vi "0036-Sub_save2.vi"   [LabVIEW 2014]
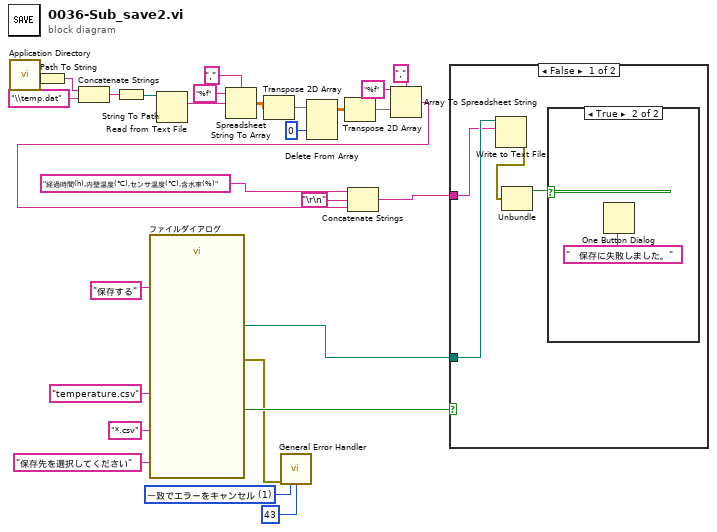
[diagram p0: block diagram]
diagram:
  w10 = 1 items=["例外なし", "一致でエラーをキャンセル", "一致でエラーをセット"] ("[exception action] (none:0)")
  n1 = call <vilib>:"Application Directory.vi"() -> ("Application Directory"=w2:path)
  n2 = Path To String(path=w2) -> (string=w3:string)
  n3 = Concatenate Strings(w3, "\\temp.dat" ("文字列")) -> (w4:string)
  n4 = String To Path(string=w4) -> (path=w5:path)
  n5 = call "ファイルダイアログ"("prompt"="保存先を選択してください", "button label"="保存する", "default name"="temperature.csv", "pattern (all files)"="*.csv") -> ("selected path"=w13:path, "cancelled"=w14:bool, "error out"=w12:errorcluster)  [unwired: 8 in, 1 out]
  n6 = Read from Text File(file (use dialog)=w5) -> (text=w15:string)  [unwired: 3 in, 3 out]
  n7 = Spreadsheet String To Array(delimiter (Tab)="," ("デリミタ（タブ）"), format string="%f" ("形式文字列"), spreadsheet string=w15) -> (array=w24:dbl[][])  [unwired: 1 in]
  n8 = Transpose 2D Array(2D array=w24) -> (transposed array=w18:dbl[][])
  n9 = call <vilib>:"General Error Handler.vi"("error in (no error)"=w12, "[exception action] (none:0)"=w10, "[exception code]"=43) -> ()  [unwired: 8 in, 5 out]
  n10 = Delete From Array(array=w18, index (row)=0 ("指標 （行）")) -> (array with subset deleted=w20:dbl[][])  [unwired: 2 in, 1 out]
  n11 = Transpose 2D Array(2D array=w20) -> (transposed array=w21:dbl[][])
  n12 = Array To Spreadsheet String(delimiter (Tab)="," ("デリミタ（タブ）"), array=w21, 3:"%f" ("形式文字列")) -> (spreadsheet string=w26:string)
  n13 = Concatenate Strings("経過時間(h),内壁温度(℃),センサ温度(℃),含水率(%)", "\r\n", w26) -> (w27:string)
  n14 = case shown="FALSE" w14 {
    tunnel: w13 -> [w32 _]
    tunnel: w27 -> [w29 _]
    frame False {
      n15 = Write to Text File(file (use dialog)=w32, text=w29) -> (error out=w31:errorcluster)  [unwired: 2 in, 2 out]
      n16 = Unbundle(w31) -> ("status"=w30:bool)  [unwired: 2 out]
      n17 = case shown="TRUE" w30 {
        frame False {
        }
        frame True {
          n18 = One Button Dialog(message="　保存に失敗しました。" ("メッセージ")) -> ()  [unwired: 1 in, 1 out]
        }
      }
    }
    frame True {
    }
  }
